vi "Verify Font Name and Size.vi"(10 "Font IN":T1={"Name"="", "Size"=-1.0, "Color"=0, "Style"={"Bold"=FALSE, "Italic"=FALSE, "Underline"=FALSE, "Strikeout"=FALSE}}, 11 "Default Font cluster":T1={"Name"="Helvetica", "Size"=12.0, "Color"=0, "Style"={"Bold"=FALSE, "Italic"=FALSE, "Underline"=FALSE, "Strikeout"=FALSE}}) -> (2 "Font OUT":T1={"Name"="Helvetica", "Size"=12.0, "Color"=0, "Style"={"Bold"=FALSE, "Italic"=FALSE, "Underline"=FALSE, "Strikeout"=FALSE}}, 3 "Font = default font":bool)   [LabVIEW 2012]
doc: "Version 1.0\nDeveloped by Jean-Marc Simard\nCopyright © 2010, Exaprom Inc.\nAll rights reserved.\nLicense: BSD"
uses:
  Controls/Font cluster.ctl
  Controls/Font size.ctl
  Controls/Font color.ctl
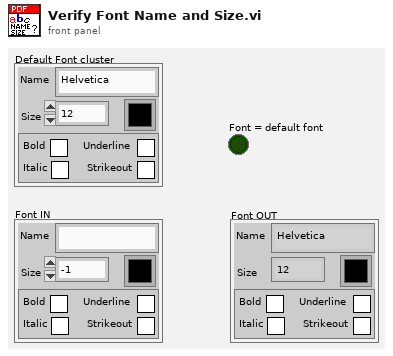
[diagram p1: front panel]
types:
  T1 = typedef "Font cluster.ctl" = cluster{"Name":string, "Size":T2, "Color":T3, "Style":cluster{"Bold":bool, "Italic":bool, "Underline":bool, "Strikeout":bool}}
  T2 = typedef "Font size.ctl" = sgl
  T3 = typedef "Font color.ctl" = u32
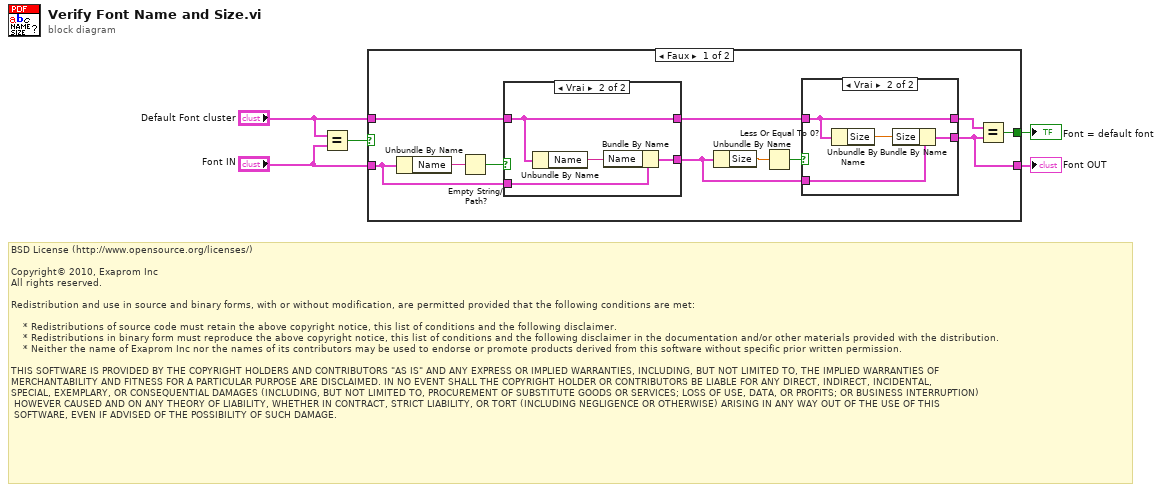
[diagram p0: block diagram]
diagram:
  # "BSD License (http://www.opensource.org/licenses/)\n\nCopyright© 2010, Exaprom Inc\nAll rights reserved.\n\nRedistribution and use in source and binary forms, with or without modification, are permitted provided that the following conditions are met:\n\n    * Redistributions of source code must retain the above copyright notice, this list of conditions and the following disclaimer.\n    * Redistributions in binary form must reproduce the above copyright notice, this list of conditions and the following disclaimer in the documentation and/or other materials provided with the distribution.\n    * Neither the name of Exaprom Inc nor the names of its contributors may be used to endorse or promote products derived from this software without specific prior written permission.\n\nTHIS SOFTWARE IS PROVIDED BY THE COPYRIGHT HOLDERS AND CONTRIBUTORS \"AS IS\" AND ANY EXPRESS OR IMPLIED WARRANTIES, INCLUDING, BUT NOT LIMITED TO, THE IMPLIED WARRANTIES OF \nMERCHANTABILITY AND FITNESS FOR A PARTICULAR PURPOSE ARE DISCLAIMED. IN NO EVENT SHALL THE COPYRIGHT HOLDER OR CONTRIBUTORS BE LIABLE FOR ANY DIRECT, INDIRECT, INCIDENTAL,\nSPECIAL, EXEMPLARY, OR CONSEQUENTIAL DAMAGES (INCLUDING, BUT NOT LIMITED TO, PROCUREMENT OF SUBSTITUTE GOODS OR SERVICES; LOSS OF USE, DATA, OR PROFITS; OR BUSINESS INTERRUPTION)\n HOWEVER CAUSED AND ON ANY THEORY OF LIABILITY, WHETHER IN CONTRACT, STRICT LIABILITY, OR TORT (INCLUDING NEGLIGENCE OR OTHERWISE) ARISING IN ANY WAY OUT OF THE USE OF THIS\n SOFTWARE, EVEN IF ADVISED OF THE POSSIBILITY OF SUCH DAMAGE."
  n1 = Equal?(x="Default Font cluster", y="Font IN") -> (x = y?=w5:bool)
  n2 = case shown="Faux" w5 {
    selector: w5 -> [_ w30]
    tunnel: "Default Font cluster" -> [w13 _]
    tunnel: "Font IN" -> [w14 w29]
    tunnel: [w7 w30] -> w2
    tunnel: [w6 w29] -> w1
    frame False {
      n3 = Unbundle By Name(w14) -> ("Name"=w16:string)
      n4 = Empty String/Path?(string/path=w16) -> (empty?=w15:bool)
      n5 = case shown="Vrai" w15 {
        tunnel: w14 -> [w24 w27]
        tunnel: w13 -> [w23 w25]
        tunnel: [w24 w26] -> w10
        tunnel: [w23 w25] -> w9
        frame False {
        }
        frame True {
          n6 = Unbundle By Name(w25) -> ("Name"=w28:string)
          n7 = Bundle By Name(cluster=w27, "Name"=w28) -> (w26:T1)
        }
      }
      n8 = Unbundle By Name(w10) -> ("Size"=w12:T2)
      n9 = Less Or Equal To 0?(x=w12) -> (x <= 0?=w11:bool)
      n10 = case shown="Vrai" w11 {
        tunnel: w10 -> [w18 w22]
        tunnel: w9 -> [w17 w19]
        tunnel: [w18 w20] -> w6
        tunnel: [w17 w19] -> w8
        frame False {
        }
        frame True {
          n11 = Unbundle By Name(w19) -> ("Size"=w21:T2)
          n12 = Bundle By Name(cluster=w22, "Size"=w21) -> (w20:T1)
        }
      }
      n13 = Equal?(x=w8, y=w6) -> (x = y?=w7:bool)
    }
    frame True {
    }
  }
  "Font = default font" <- w2
  "Font OUT" <- w1
